vi "Clear Tools.vi"(8 "error in":errorcluster, 11 "id":i32) -> (0 "error in 2":errorcluster, 3 "id out":i32)   [LabVIEW 2025, in "MCP Server.lvlib"]
doc: "Deletes all tools from a MCP server."
uses:
  MCP Server.lvlib
  Tool Data.ctl
  Input Parameter.ctl
  Output Parameter.ctl
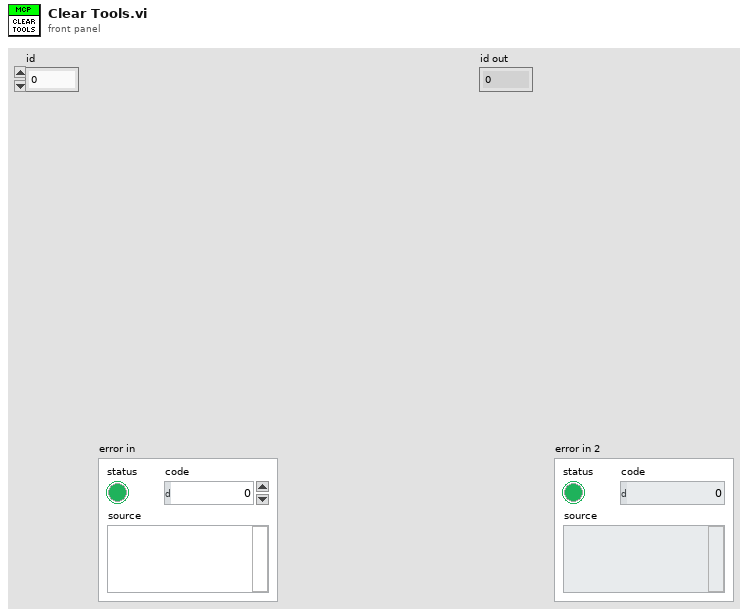
[diagram p1: front panel]
types:
  T1 = typedef "MCP Server.lvlib/Tool Data.ctl" = cluster{"Name":string, "Description":string, "Ignored":string[], "inputs":T2[], "outputs":T3[], "VI Refnum":refnum<vi>}
  T2 = typedef "MCP Server.lvlib/Input Parameter.ctl" = cluster{"name":string, "type":string, "description":string, "required":bool, "raw name":string}
  T3 = typedef "MCP Server.lvlib/Output Parameter.ctl" = cluster{"name":string, "description":string, "type":string, "raw name":string}
  T4 = typedef "MCP Server.lvlib/Server Data.ctl" = cluster{"Name":string, "Description":string, "Tools":T1[], "Parameters":string[][], "Logging Info":T5, "User Events":T6, "Prompts":T7[], "resources":T9[], "HTTP Server":refnum<class "Server.lvclass">}
  T5 = typedef "MCP Server.lvlib/Logging.ctl" = cluster{"Log":string[], "Max Length":i32}
  T6 = typedef "MCP Server.lvlib/User Events.ctl" = cluster{"onError":refnum<user-event>, "onRpc":refnum<user-event>}
  T7 = typedef "MCP Server.lvlib/Prompt Data.ctl" = cluster{"name":string, "description":string, "arguments":T8[], "return terminal name":string, "results description":string, "VI Refnum":refnum<vi>}
  T8 = typedef "MCP Server.lvlib/Prompt Argument.ctl" = cluster{"name":string, "description":string, "required":bool, "raw_name":string}
  T9 = typedef "MCP Server.lvlib/resource data.ctl" = cluster{"uri":string, "name":string, "description":string, "mimeType":string, "file path":path}
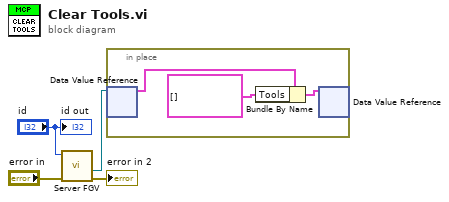
[diagram p0: block diagram]
diagram:
  n1 = call "Server FGV.vi"("error in"="error in", "id"="id") -> ("error out"=→"error in 2":errorcluster, "server reference"=w1:refnum<data-value>)  [unwired: 5 in, 3 out]
  n2 = in-place {
    n3 = in-place-dvr #1(w1) -> (w7:T4)  [unwired: 1 out]
    n4 = Bundle By Name(cluster=w7, "Tools"=T1[] []) -> (w6:T4)
    n5 = in-place-dvr #1(w6) -> ()  [unwired: 2 out]
  }
  "id out" <- "id"
